vi "1L26_mesure_resistance.vi"(1 "I ref":dbl, 2 "Vref":dbl, 3 "Rc":dbl, 4 "Vm":dbl) -> (0 "Rm":dbl)   [LabVIEW 2010, in "lv_01.lvlib"]
doc: "Vm est la tension aux bornes de Rm\nSi Rc=0 alors Rm est calculé selon iref, sinon, Vref alimente Rc et Rm en série"
uses:
  lv_01.lvlib
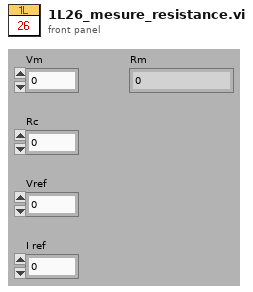
[diagram p1: front panel]
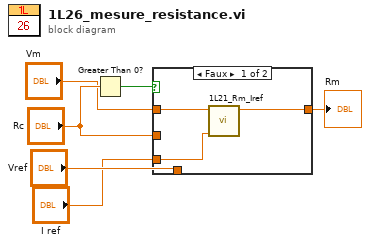
[diagram p0: block diagram]
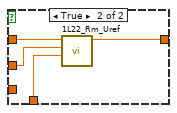
[diagram p2: hidden frame]
diagram:
  n1 = Greater Than 0?(x="Rc") -> (x > 0?=w3:bool)
  n2 = case shown="Faux" w3 {
    tunnel: "Vm" -> [w8 w13]
    tunnel: "Rc" -> [_ w12]
    tunnel: [w9 w11] -> w4
    tunnel: "I ref" -> [w7 _]
    tunnel: "Vref" -> [_ w10]
    frame False {
      n3 = call "1L21_Rm_Iref.vi"("I ref"=w7, "Vm"=w8) -> ("Rm"=w9:dbl)  [unwired: 9 in]
    }
    frame True {
      n4 = call "1L22_Rm_Uref.vi"("Uref"=w10, "Rc"=w12, "Um"=w13) -> ("Rm"=w11:dbl)  [unwired: 8 in]
    }
  }
  "Rm" <- w4
